vi "Maxi Gauge-Net-Connect.vi"(8 "Fehler (Eingang)":errorcluster, 9 "stop":bool, 10 "Baud Rate":u16(ring)=4 items=["300", "1200", "2400", "4800", "9600", "19200"], 11 "VISA-Ressource in":refnum<visa-resource-name>) -> (0 "Fehler (Ausgang)":errorcluster, 1 "Connection":bool[](array[boolean]), 2 "Net-Numbers":u8[](array[numeric]), 3 "VISA-Ressource out":refnum<visa-resource-name>, 5 "Actual Net-Number":u8)   [LabVIEW 2012, in "Maxi Gauge.lvlib"]
uses:
  Maxi Gauge.lvlib
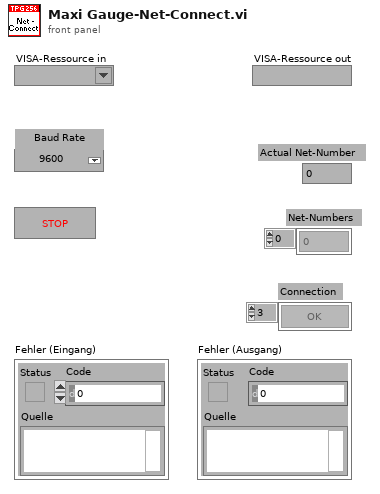
[diagram p1: front panel]
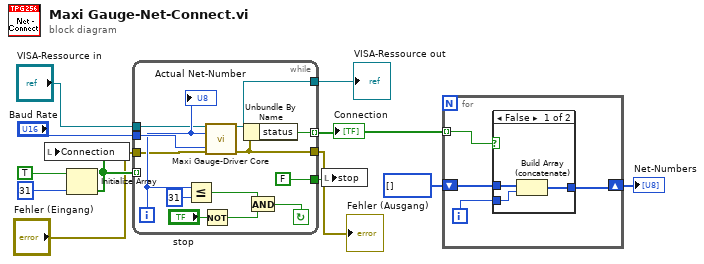
[diagram p0: block diagram]
diagram:
  n1 = Initialize Array(TRUE, 31) -> (w9:bool[])
  n2 = local write "Connection"(w9) -> ()
  n3 = while {
    tunnel: [FALSE] -> w8
    tunnel: w9 -> [_] mode=indexing
    tunnel: [w13] -> w7 mode=indexing
    tunnel: "Baud Rate" -> [w25]
    tunnel: "VISA-Ressource in" -> [w17]
    tunnel: [w16] -> w3
    tunnel: "Fehler (Eingang)" -> [w15]
    tunnel: [w14] -> w1
    i -> [w18]
    stop <- w20 continue-if-true
    n4 = Less Or Equal?(x=w18, y=31) -> (x <= y?=w23:bool)
    n5 = Not(x="stop") -> (.not. x?=w21:bool)
    n6 = call "Maxi Gauge-Driver Core.vi"("VISA-Ressource in"=w17, "Node address"=w18, "Fehler (Eingang)"=w15, "Timeout [ms]"=w25) -> ("VISA-Ressource out"=w16:refnum<visa-resource-name>, "Fehler (Ausgang)"=w14:errorcluster)  [unwired: 9 in, 1 out]
    n7 = Unbundle By Name(w14) -> ("status"=w13:bool)
    n8 = And(x=w23, y=w21) -> (x .and. y?=w20:bool)
    "Actual Net-Number" <- w18
  }
  "Connection" <- w7
  "VISA-Ressource out" <- w3
  "Fehler (Ausgang)" <- w1
  n9 = local write "stop"(w8) -> ()
  n10 = for {
    tunnel: w7 -> [w29] mode=indexing
    shift-right: [w26] -> w6
    shift-left: i32[] [] -> [w28]
    i -> [w27]
    n11 = case shown="False" w29 {
      tunnel: w28 -> [w32 w33]
      tunnel: w27 -> [w31 _]
      tunnel: [w30 w33] -> w26
      frame False {
        n12 = Build Array (concatenate)(w32, w31) -> (w30:i32[])
      }
      frame True {
      }
    }
  }
  "Net-Numbers" <- w6
